vi "main_WS2.vi"() -> ()   [LabVIEW 2017]
uses:
  <vilib>/Instr/_visa.llb/VISA Configure Serial Port (Instr).vi
panel:
  out "validFix":string
  out "validHDOP":dbl
  out "validaltitude [m]":dbl
  out "validdate":string
  out "validSpeed [Knots]":dbl
  out "validE/W":string
  out "validlong":string
  out "validN/S":string
  out "validLat":string
  out "UTC+2":timestamp format="%<%.3X>T"
  out "Lat 2":string caption="Latitude"
  out "tVOC":dbl
  out "CO2":dbl
  out "Temperature":dbl
  out "Altitude":dbl
  out "Pressure":dbl
  out "Humidity":dbl
  in  "Start/Stop Map":bool
  out "NumericLong":dbl
  out "NumericLat":dbl
  in  "Zoom":i32(slide)=6 scale=0.0..21.0
  in  "Map type":string(combo)="roadmap"
  out "URL":string
  in  "Refresh rate [ms]":u32=1000 step=1000
  in  "?":refnum<k7>(container)
  out "Err Msg":string
  out "Rain":bool
  out "WindDir":dbl
  out "WindSpeed":dbl
  out "Fix String":string
  out "Status2":bool
  out "UTC 2":string
  out "Status":string
  out "N/S 2":string caption="N/S"
  out "long 2":string caption="Longitude"
  out "E/W 2":string caption="E/W"
  out "date":string
  out "Speed [Knots]":dbl
  out "Track angle degrees":dbl
  out "output 10":string
  out "UTC time":string
  out "Latitude":string
  out "N/S":string
  out "Longitude":string
  out "E/W":string
  out "Fix":string
  out "Satellites used":string
  out "HDOP":dbl
  out "altitude [m]":dbl
  in  "Reconnect":bool
  out "read buffer":string
  in  "Exit":bool
  in  "baud rate":u32=57600
  in  "VISA resource name":refnum<visa-resource-name>="COM1"
  # "Weather Station"
  # "GPS"
  # "Wind Speed"
  # "Rain"
  # "Km/hr"
  # "Wind Direction"
  # "degree"
  # "BME"
  # "Air Quality"
  # "%"
  # "Pa"
  # "m"
  # "C"
  # "Communication:"
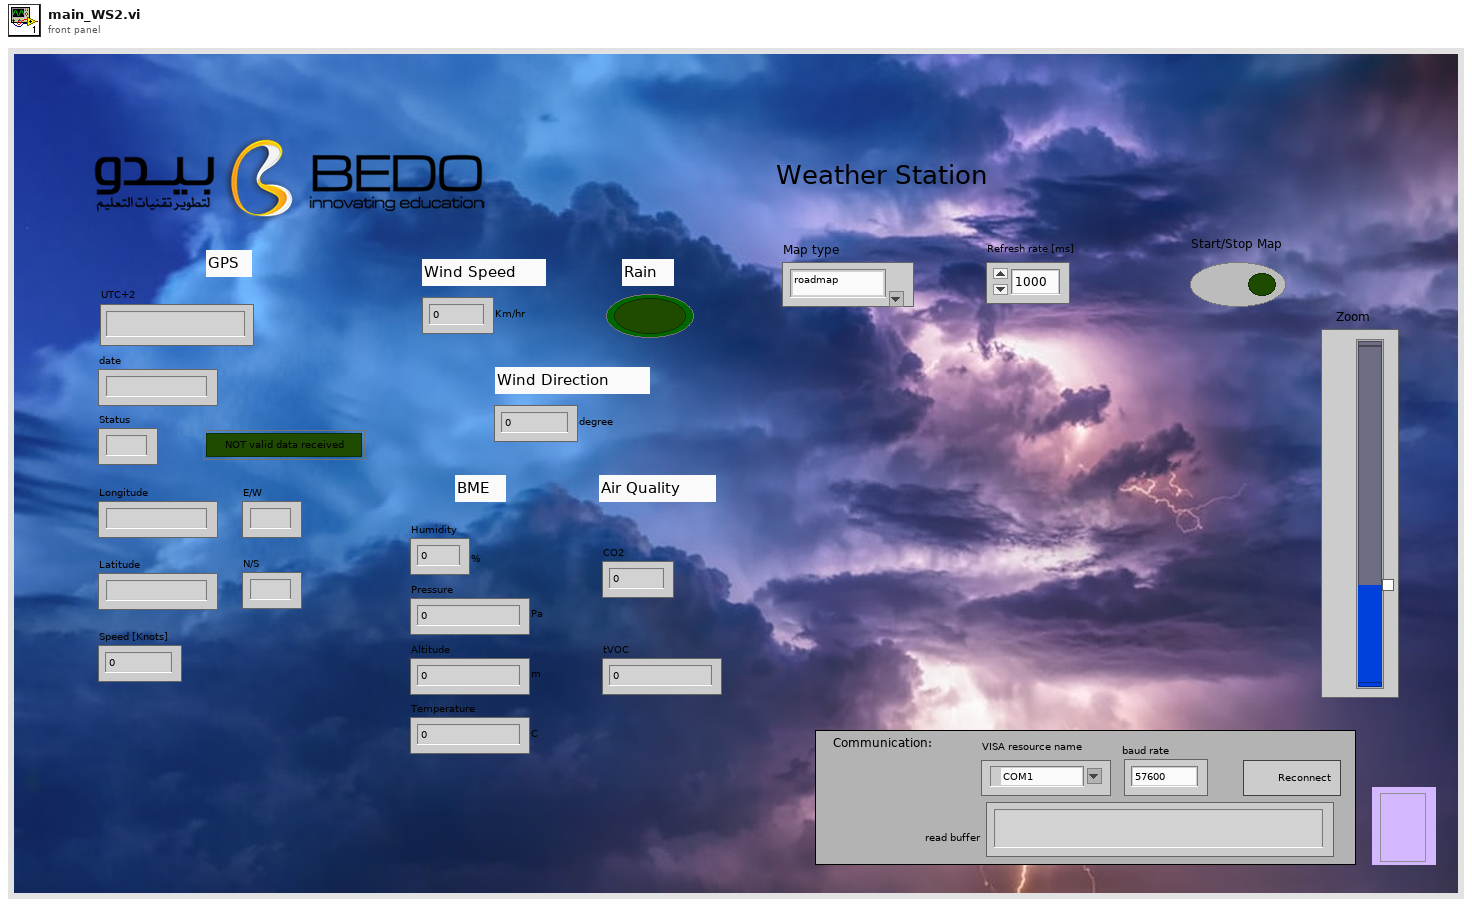
[diagram p1: front panel]
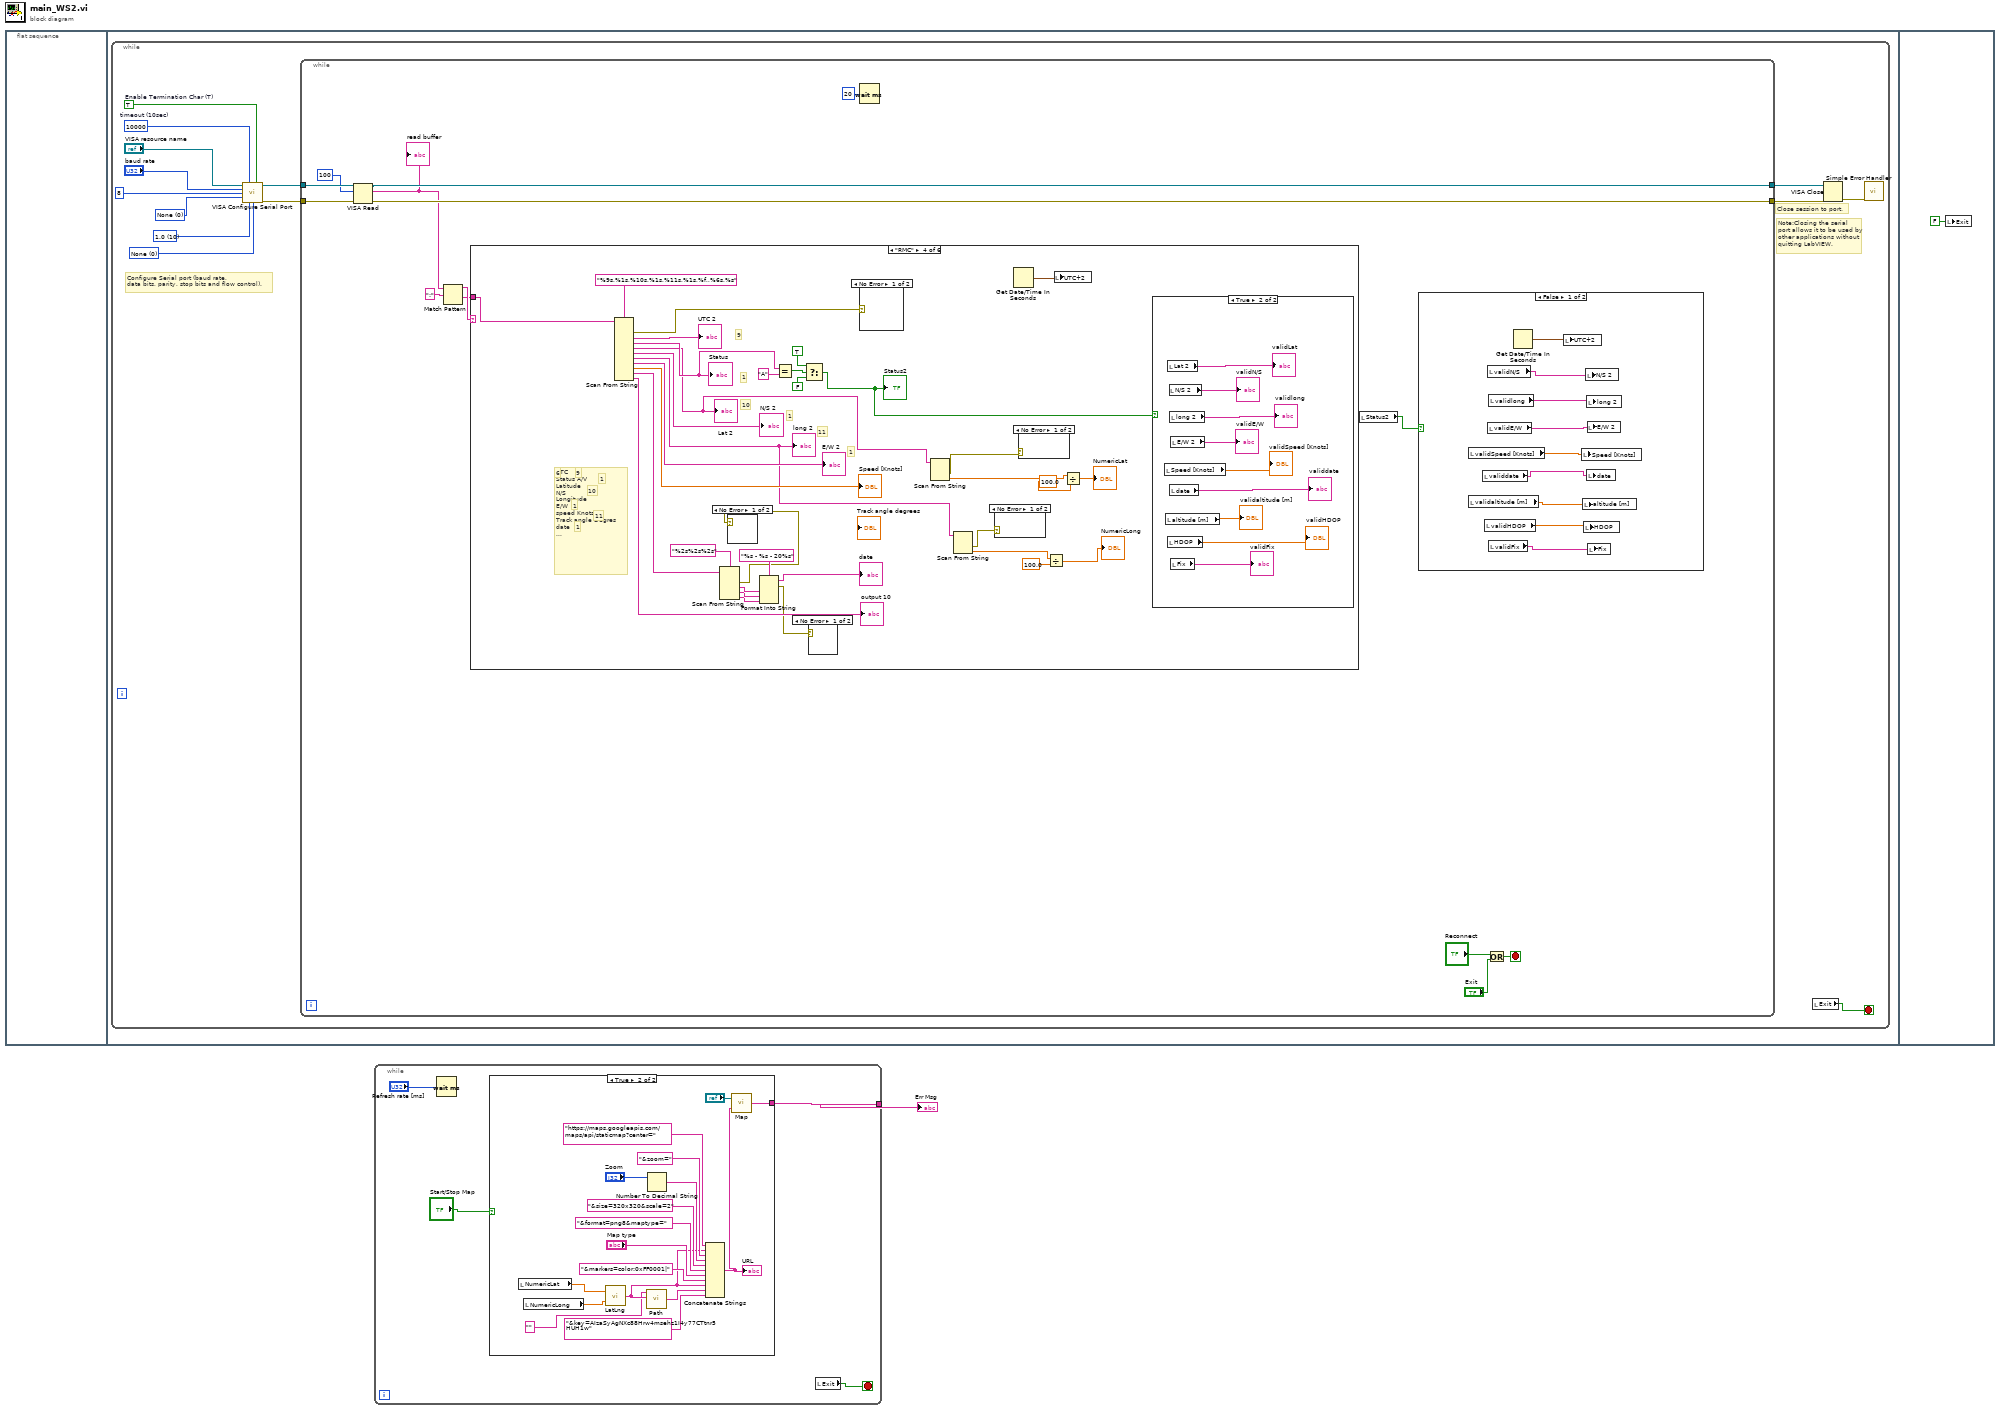
[diagram p0: block diagram]
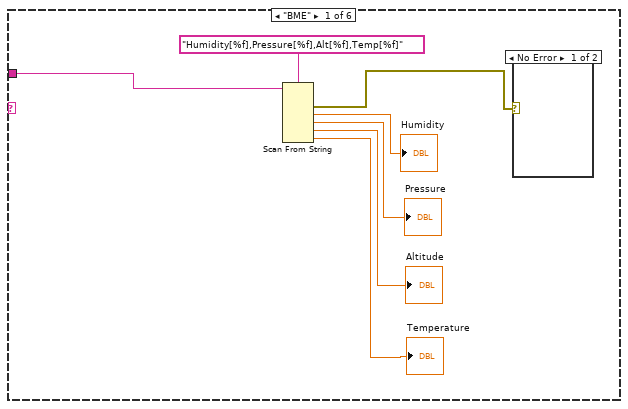
[diagram p4: hidden frame]
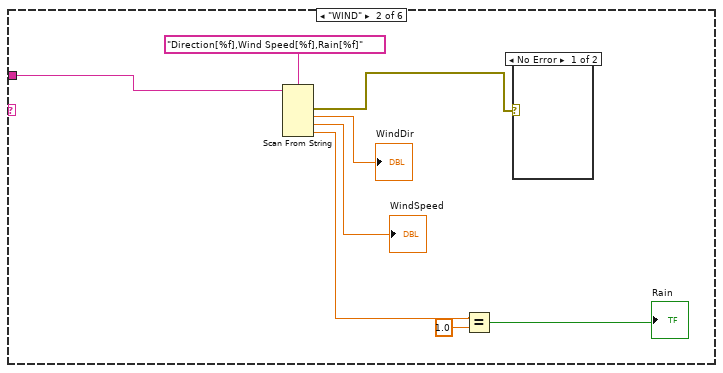
[diagram p6: hidden frame]
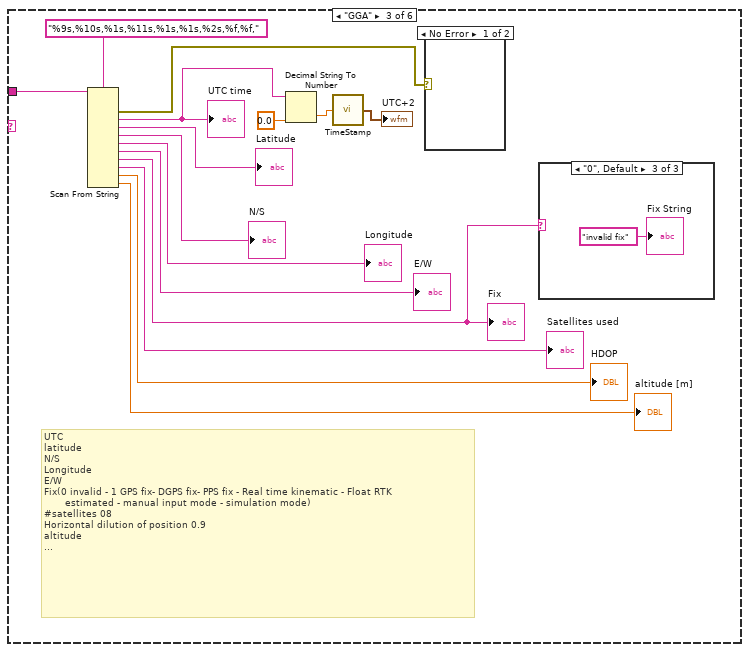
[diagram p8: hidden frame]
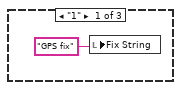
[diagram p9: hidden frame]
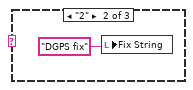
[diagram p10: hidden frame]
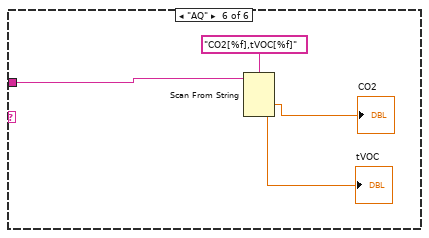
[diagram p19: hidden frame]
diagram:
  n1 = flat-sequence {
    frame #0 {
    }
    frame #1 {
      n2 = while {
        stop <- w2 stop-if-true
        w14 = u16 0 items=["None"=0, "XON/XOFF"=1, "RTS/CTS"=2, "DTR/DSR"=4] ("flow control")
        w13 = u16 10 items=["1.0"=10, "1.5"=15, "2.0"=20] ("stop bits")
        w10 = u16 0 items=["None", "Odd", "Even", "Mark", "Space"] ("parity")
        w12 = TRUE  # Enable Termination Char (T)
        w11 = u32 10000  # timeout (10sec)
        # "Note:Closing the serial port allows it to be used by other applications without\nquitting LabVIEW."
        # "Close session to port."
        # "Configure Serial port (baud rate,\ndata bits, parity, stop bits and flow control)."
        n3 = call-poly "VISA Configure Serial Port"("VISA resource name"="VISA resource name", "timeout (10sec)"=w11, "Enable Termination\nChar (T)"=w12, "baud rate (9600)"="baud rate", "data bits (8)"=u16 8 ("data bits"), "parity (0:none)"=w10, "stop bits (10: 1 bit)"=w13, "flow control (0:none)"=w14) -> ("VISA resource name out"=w7:refnum<visa-resource-name>, "error out"=w6:errorcluster)  [unwired: 6 in]
        n4 = while {
          tunnel: w7 -> [w29]
          tunnel: w6 -> [w28]
          tunnel: [w26] -> w4
          tunnel: [w25] -> w3
          stop <- w17 stop-if-true
          n5 = VISA Read(VISA resource name=w29, byte count=u32 100, error in (no error)=w28) -> (VISA resource name out=w25:refnum<visa-resource-name>, read buffer=w21:string, error out=w26:errorcluster)  [unwired: 1 out]
          "read buffer" <- w21
          n6 = Match Pattern(string=w21, regular expression=":") -> (before substring=w23:string, after substring=w22:string)  [unwired: 1 in, 2 out]
          n7 = case shown="\"RMC\"" w23 {
            tunnel: w22 -> [w44 w52 w60 w98 _ w118]
            frame "BME" {
              n8 = Scan From String(format string="Humidity[%f],Pressure[%f],Alt[%f],Temp[%f]", input string=w44) -> (error out=w43:errorcluster, output 1=→"Humidity":dbl, output 2=→"Pressure":dbl, output 3=→"Altitude":dbl, output 4=→"Temperature":dbl)  [unwired: 6 in, 2 out]
              n9 = case shown="No Error" w43 {
                frame No Error {
                }
                frame Error {
                }
              }
            }
            frame "WIND" {
              n10 = Scan From String(format string="Direction[%f],Wind Speed[%f],Rain[%f]", input string=w52) -> (error out=w51:errorcluster, output 1=→"WindDir":dbl, output 2=→"WindSpeed":dbl, output 3=w48:dbl)  [unwired: 5 in, 2 out]
              n11 = Equal?(x=w48, y=1.0) -> (x = y?=→"Rain":bool)
              n12 = case shown="No Error" w51 {
                frame No Error {
                }
                frame Error {
                }
              }
            }
            frame "GGA" {
              # "UTC\nlatitude\nN/S\nLongitude\nE/W\nFix(0 invalid - 1 GPS fix- DGPS fix- PPS fix - Real time kinematic - Float RTK\n       estimated - manual input mode - simulation mode)\n#satellites 08\nHorizontal dilution of position 0.9\naltitude\n..."
              n13 = Scan From String(format string="%9s,%10s,%1s,%11s,%1s,%1s,%2s,%f,%f,", input string=w60) -> (error out=w63:errorcluster, output 1=w54:string, output 2=→"Latitude":string, output 3=→"N/S":string, output 4=→"Longitude":string, output 5=→"E/W":string, output 6=w61:string, output 7=→"Satellites used":string, output 8=→"HDOP":dbl, output 9=→"altitude [m]":dbl)  [unwired: 11 in, 2 out]
              "UTC time" <- w54
              "Fix" <- w61
              n14 = Decimal String To Number(string=w54, default (0L)=0.0 ("default (0 I32)")) -> (number=w56:dbl)  [unwired: 1 in, 1 out]
              n15 = call "TimeStamp.vi"("Numeric Indicator"=w56) -> ("Time Stamp Control"=→"UTC+2":timestamp)
              n16 = case shown="No Error" w63 {
                frame No Error {
                }
                frame Error {
                }
              }
              n17 = case shown="\"0\", Default" w61 {
                frame "1" {
                  n18 = local write "Fix String"("GPS fix" ("Fix String")) -> ()
                }
                frame "2" {
                  n19 = local write "Fix String"("DGPS fix" ("Fix String")) -> ()
                }
                frame "0", Default {
                  "Fix String" <- "invalid fix" ("Fix String")
                }
              }
            }
            frame "RMC" {
              # "6"
              # "1"
              # "11"
              # "1"
              # "10"
              # "1"
              # "9"
              # "1"
              # "11"
              # "1"
              # "10"
              # "1"
              # "9"
              # "UTC\nStatus A/V\nLatitude\nN/S\nLongitude\nE/W\nspeed Knots\nTrack angle Degres\ndate\n..."
              n20 = Scan From String(format string="%9s,%1s,%10s,%1s,%11s,%1s,%f,,%6s,%s", input string=w98) -> (error out=w100:errorcluster, output 1=→"UTC 2":string, output 2=w96:string, output 3=w79:string, output 4=→"N/S 2":string, output 5=w74:string, output 6=→"E/W 2":string, output 7=→"Speed [Knots]":dbl, output 8=w90:string, output 9=→"output 10":string)  [unwired: 11 in, 2 out]
              "Status" <- w96
              "Lat 2" <- w79
              "long 2" <- w74
              n21 = Scan From String(format string="%2s%2s%2s", input string=w90) -> (error out=w73:errorcluster, output 1=w88:string, output 2=w87:string, output 3=w86:string)  [unwired: 5 in, 2 out]
              n22 = case shown="No Error" w73 {
                frame No Error {
                }
                frame Error {
                }
              }
              n23 = Format Into String(format string="%s - %s - 20%s", w88, w87, w86) -> (resulting string=→"date":string, error out=w72:errorcluster)  [unwired: 2 in]
              n24 = Equal?(x=w96, y="A") -> (x = y?=w97:bool)
              n25 = Select(t=TRUE, s=w97, f=FALSE) -> (s? t:f=w92:bool)
              "Status2" <- w92
              n26 = case shown="No Error" w72 {
                frame No Error {
                }
                frame Error {
                }
              }
              n27 = case shown="No Error" w100 {
                frame No Error {
                }
                frame Error {
                }
              }
              n28 = Scan From String(input string=w79) -> (error out=w81:errorcluster, output 1=w82:dbl)  [unwired: 4 in, 2 out]
              n29 = Scan From String(input string=w74) -> (error out=w76:errorcluster, output 1=w78:dbl)  [unwired: 4 in, 2 out]
              n30 = case shown="No Error" w76 {
                frame No Error {
                }
                frame Error {
                }
              }
              n31 = Get Date/Time In Seconds() -> (seconds since 1Jan1904=w91:timestamp)
              n32 = case shown="No Error" w81 {
                frame No Error {
                }
                frame Error {
                }
              }
              n33 = Divide(x=w78, y=100.0) -> (x/y=→"NumericLong":dbl)
              n34 = local write "UTC+2"(w91) -> ()
              n35 = Divide(x=w82, y=100.0) -> (x/y=→"NumericLat":dbl)
              n36 = case shown="True" w92 {
                frame False {
                }
                frame True {
                  n37 = local read "Speed [Knots]"() -> (→"validSpeed [Knots]":dbl)
                  n38 = local read "altitude [m]"() -> (→"validaltitude [m]":dbl)
                  n39 = local read "HDOP"() -> (→"validHDOP":dbl)
                  n40 = local read "Lat 2"() -> (→"validLat":string)
                  n41 = local read "N/S 2"() -> (→"validN/S":string)
                  n42 = local read "long 2"() -> (→"validlong":string)
                  n43 = local read "date"() -> (→"validdate":string)
                  n44 = local read "E/W 2"() -> (→"validE/W":string)
                  n45 = local read "Fix"() -> (→"validFix":string)
                }
              }
            }
            frame Default {
            }
            frame "AQ" {
              n46 = Scan From String(format string="CO2[%f],tVOC[%f]", input string=w118) -> (output 1=→"CO2":dbl, output 2=→"tVOC":dbl)  [unwired: 4 in, 3 out]
            }
          }
          n47 = Wait (ms)(milliseconds to wait=u32 20) -> ()  [unwired: 1 out]
          n48 = local read "Status2"() -> (w16:bool)
          n49 = case shown="False" w16 {
            frame False {
              n50 = local read "validSpeed [Knots]"() -> (w34:dbl)
              n51 = local read "validaltitude [m]"() -> (w32:dbl)
              n52 = local read "validdate"() -> (w33:string)
              n53 = local read "validHDOP"() -> (w31:dbl)
              n54 = local read "validN/S"() -> (w37:string)
              n55 = local read "validE/W"() -> (w35:string)
              n56 = local read "validlong"() -> (w36:string)
              n57 = local read "validFix"() -> (w30:string)
              n58 = Get Date/Time In Seconds() -> (seconds since 1Jan1904=w38:timestamp)
              n59 = local write "UTC+2"(w38) -> ()
              n60 = local write "Speed [Knots]"(w34) -> ()
              n61 = local write "altitude [m]"(w32) -> ()
              n62 = local write "HDOP"(w31) -> ()
              n63 = local write "N/S 2"(w37) -> ()
              n64 = local write "long 2"(w36) -> ()
              n65 = local write "date"(w33) -> ()
              n66 = local write "E/W 2"(w35) -> ()
              n67 = local write "Fix"(w30) -> ()
            }
            frame True {
            }
          }
          n68 = Or(x="Reconnect", y="Exit") -> (x .or. y?=w17:bool)
        }
        n69 = local read "Exit"() -> (w2:bool)
        n70 = VISA Close(VISA resource name=w3, error in (no error)=w4) -> (error out=w5:errorcluster)
        n71 = call <vilib>:"Simple Error Handler.vi"("error in (no error)"=w5) -> ()  [unwired: 4 in, 5 out]
      }
    }
    frame #2 {
      n72 = local write "Exit"(FALSE ("Exit")) -> ()
    }
  }
  n73 = while {
    tunnel: [w123] -> w1
    stop <- w120 stop-if-true
    n74 = Wait (ms)(milliseconds to wait="Refresh rate [ms]") -> ()  [unwired: 1 out]
    n75 = case shown="True" "Start/Stop Map" {
      tunnel: [_ w140] -> w123
      frame False {
      }
      frame True {
        n76 = local read "NumericLat"() -> (w126:dbl)
        n77 = local read "NumericLong"() -> (w125:dbl)
        n78 = call "LatLng.vi"("Longitude"=w125, "Latitude"=w126) -> ("<Lat>,<Lng>"=w128:string)
        n79 = call "Path.vi"("End Lat,Lng"=w128, "Start Lat,Lng"="") -> ("Path"=w131:string)  [unwired: 2 in]
        n80 = Number To Decimal String(number="Zoom") -> (decimal integer string=w136:string)  [unwired: 1 in]
        n81 = Concatenate Strings("https://maps.googleapis.com/maps/api/staticmap?center=" ("string"), w128, "&zoom=" ("string"), w136, "&size=320x320&scale=2" ("string"), "&format=png8&maptype=" ("string"), "Map type", "&markers=color:0xFF0001|", w128, w131, "&key=AIzaSyAgNXc88Hrw4msehz1I4y77CTtnr5HUH1w" ("string")) -> (w127:string)
        "URL" <- w127
        n82 = call "Map.vi"("URL"=w127, "WebBrowser"="?") -> ("Error Msg"=w140:string)
      }
    }
    n83 = local read "Exit"() -> (w120:bool)
  }
  "Err Msg" <- w1
